vi "fgRptEna.vi"(7 "eRptType":T2(ring)=enum."Clear", 11 "rdoTest Type":T1) -> (3 "ENA":T3(ring))   [LabVIEW 2014]
uses:
  typedef/rdoTestType.ctl
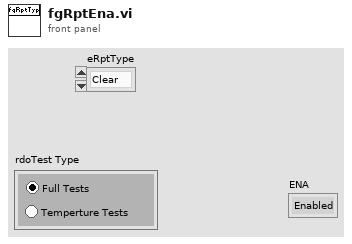
[diagram p1: front panel]
types:
  T1 = typedef "rdoTestType.ctl" = enum32{"rFull", "rTemp"}
  T2 = enum16{"get", "Clear", "Set Temp", "Set PFI", "Set Step"}
  T3 = enum8{"Enabled", "Disabled", "Disabled and Grayed Out"}
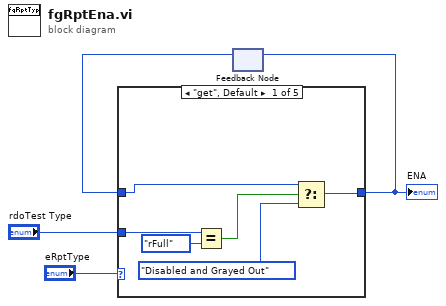
[diagram p0: block diagram]
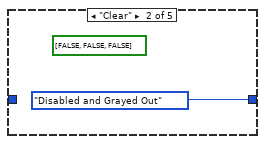
[diagram p2: hidden frame]
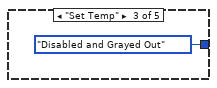
[diagram p3: hidden frame]
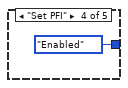
[diagram p4: hidden frame]
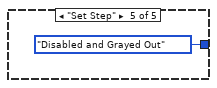
[diagram p5: hidden frame]
diagram:
  n1 = feedback #1() -> (w2:T3)  [unwired: 1 in]
  n2 = case shown="\"get\", Default" "eRptType" {
    tunnel: [w8 T3."Disabled and Grayed Out" ("ENA 2") T3."Disabled and Grayed Out" ("ENA 2") T3."Enabled" ("ENA 2") T3."Disabled and Grayed Out" ("ENA 2")] -> w3
    tunnel: w2 -> [w7 _ _ _ _]
    tunnel: "rdoTest Type" -> [w10 _ _ _ _]
    frame "get", Default {
      n3 = Equal?(x=w10, y=rdoTestType."rFull") -> (x = y?=w6:bool)
      n4 = Select(t=w7, s=w6, f=T3."Disabled and Grayed Out") -> (s? t:f=w8:T3)
    }
    frame "Clear" {
      (unwired) bool[] [FALSE, FALSE, FALSE]
    }
    frame "Set Temp" {
    }
    frame "Set PFI" {
    }
    frame "Set Step" {
    }
  }
  "ENA" <- w3
  n5 = feedback-in #1(w3) -> ()
